vi "encodeInt.vi"(8 "error in (no error)":errorcluster, 10 "Variant":variant) -> (0 "error out":errorcluster, 2 "Array":u8[](array[numeric]) format="%.0x")   [LabVIEW 2016, in "MsgPack.lvlib"]
uses:
  MsgPack.lvlib
  <vilib>/Utility/Data Type/NI_Data Type.lvlib
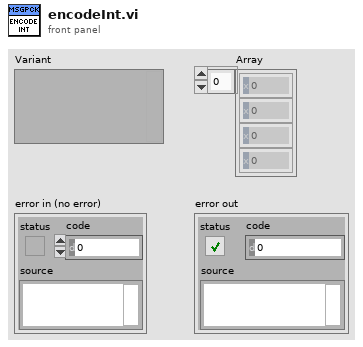
[diagram p1: front panel]
types:
  T1 = typedef "NI_Data Type.lvlib/Data Type.ctl" = enum8{"Invalid Type", "Void", "I8", "I16", "I32", "I64", "U8", "U16", "U32", "U64", "Single Float", "Double Float", "Extended Float", "Single Complex", "Double Complex", "Extended Complex", "Enum U8", "Enum U16", "Enum U32", "Enum U64", "Single Float With Unit", "Double Float With Unit", "Extended Float With Unit", "Single Complex with Unit", "Double Complex with Unit", "Extended Complex with Unit", "Boolean", "String", "Path", "Picture", "Tag", "Array", "Cluster", "Variant", "LV Variant", "Waveform", "Timestamp", "Digital Waveform", "Digital Data", "ExpressData", "Refnum", "External Data", "VI", "Poly VI", "LabVIEW Class Instance", "Fixed Point"}
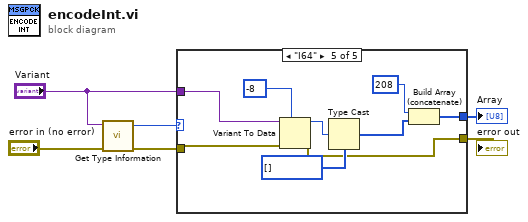
[diagram p0: block diagram]
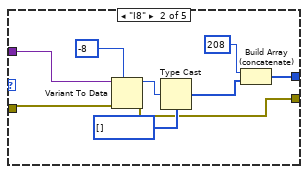
[diagram p3: hidden frame]
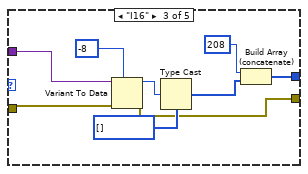
[diagram p4: hidden frame]
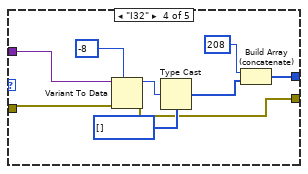
[diagram p5: hidden frame]
diagram:
  n1 = call <vilib>:"Get Type Information.vi"("error in (no error)"="error in (no error)", "Variant"="Variant") -> ("error out"=w5:errorcluster, "Type"=w6:T1)  [unwired: 5 in, 3 out]
  n2 = case shown="\"I64\"" w6 {
    tunnel: w5 -> [w7 w16 w25 w34 w43]
    tunnel: "Variant" -> [_ w15 w24 w33 w42]
    tunnel: [_ w9 w18 w27 w36] -> w3
    tunnel: [w7 w8 w17 w26 w35] -> w2
    frame "Invalid Type", Default {
    }
    frame "I8" {
      n3 = Variant To Data(error in=w16, type=i8 -8, Variant=w15) -> (data=w12:i8, error out=w8:errorcluster)
      n4 = Type Cast(type=u8[] [], x=w12) -> (*(type *) &x=w10:u8[])
      n5 = Build Array (concatenate)(u8 208, w10) -> (w9:u8[])
    }
    frame "I16" {
      n6 = Variant To Data(error in=w25, type=i16 -8, Variant=w24) -> (data=w21:i16, error out=w17:errorcluster)
      n7 = Type Cast(type=u8[] [], x=w21) -> (*(type *) &x=w19:u8[])
      n8 = Build Array (concatenate)(u8 208, w19) -> (w18:u8[])
    }
    frame "I32" {
      n9 = Variant To Data(error in=w34, type=-8, Variant=w33) -> (data=w30:i32, error out=w26:errorcluster)
      n10 = Type Cast(type=u8[] [], x=w30) -> (*(type *) &x=w28:u8[])
      n11 = Build Array (concatenate)(u8 208, w28) -> (w27:u8[])
    }
    frame "I64" {
      n12 = Variant To Data(error in=w43, type=i64 -8, Variant=w42) -> (data=w39:i64, error out=w35:errorcluster)
      n13 = Type Cast(type=u8[] [], x=w39) -> (*(type *) &x=w37:u8[])
      n14 = Build Array (concatenate)(u8 208, w37) -> (w36:u8[])
    }
  }
  "Array" <- w3
  "error out" <- w2
